vi "MGL_relativePath_cls.vi"(8 "name of main source folder [BIN]":string="BIN") -> (1 "mode":T1, 2 "Path":path)   [LabVIEW 2018]
uses:
  MGL_relativePathMode.ctl
panel:
  # "Relative Path.vi\n\nRitorna il path della directory dov'e' stato salvato, indipendentemente se chiamato da un eseguibile o no (VI di LabVIEW).\nUsando questo VI  per creare i path dei vari file utili ad un applicazione, non sarà poi necessario \nmodificare nulla creando l'eseguibile dell'applicazine.\n\nSe il VI viene salvato all'interno di directory che si trovano sotto una \"BIN\", ritornera' il path subito \"sopra\" la \"BIN\".\n - es \"C:\\app\\bin\\uno\\due\\tre\\Path.vi\"  ritornerà  \"c:\\app\"\nLo stesso vale se al posto di BIN si usano nomi che iniziano per BIN ( BINARY, BINS ...)\n\nCopyright (C) 2003 Alessandro Ricco - ale914@ilvg.it\n\n                                        Visita \"Italian LabVIEW user Group\" - www.ilvg.it\n\n\nThis library is free software; you can redistribute it and/or\nmodify it under the terms of the GNU Lesser General Public\nLicense as published by the Free Software Foundation; either\nversion 2.1 of the License, or (at your option) any later version.\nThis library is distributed in the hope that it will be useful,\nbut WITHOUT ANY WARRANTY; without even the implied warranty of\nMERCHANTABILITY or FITNESS FOR A PARTICULAR PURPOSE. See the GNU\nLesser General Public License for more details.\nYou should have received a copy of the GNU Lesser General Public\nLicense along with this library; if not, write to the Free Software\nFoundation, Inc., 59 Temple Place, Suite 330, Boston, MA 02111-1307 USA"
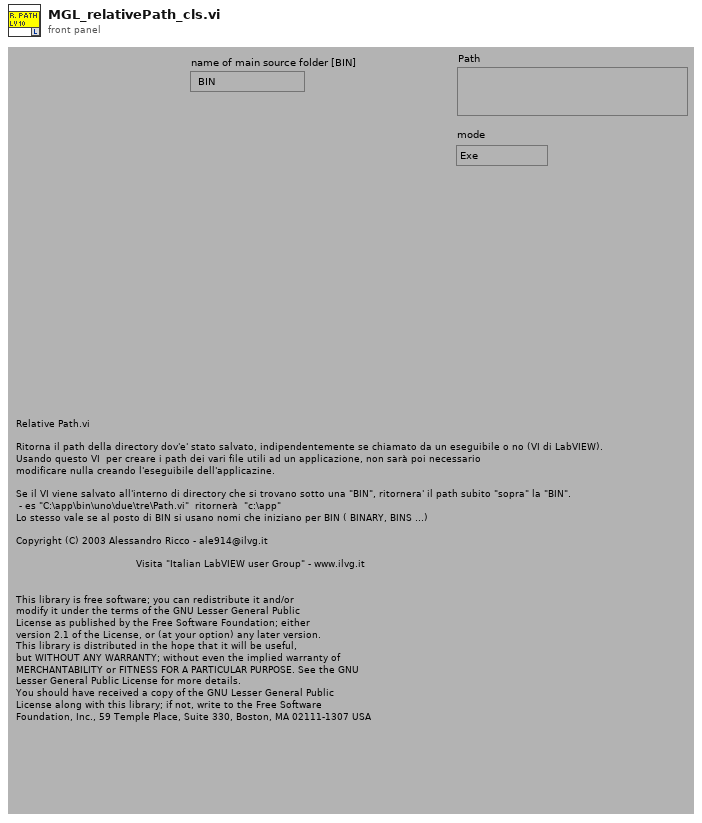
[diagram p1: front panel]
types:
  T1 = typedef "MGL_RelativePathMode.ctl" = enum16{"Exe", "LabVIEW"}
  T2 = typedef "MGL_relativePathMode.ctl" = enum16{"Exe", "LabVIEW"}
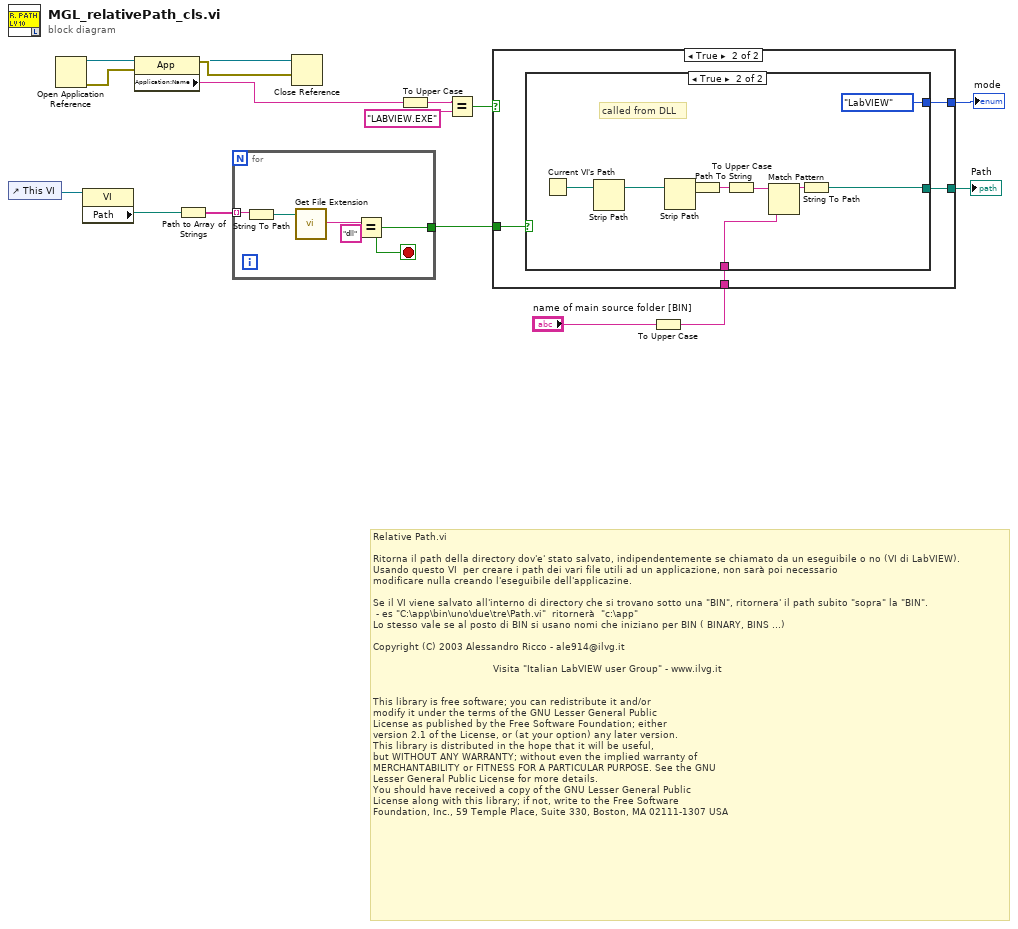
[diagram p0: block diagram]
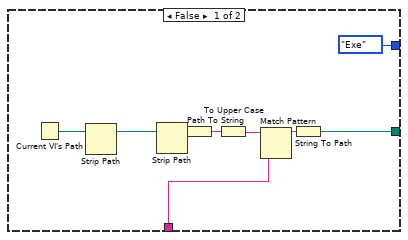
[diagram p2: hidden frame]
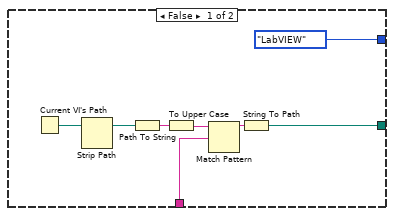
[diagram p3: hidden frame]
diagram:
  # "Relative Path.vi\n\nRitorna il path della directory dov'e' stato salvato, indipendentemente se chiamato da un eseguibile o no (VI di LabVIEW).\nUsando questo VI  per creare i path dei vari file utili ad un applicazione, non sarà poi necessario \nmodificare nulla creando l'eseguibile dell'applicazine.\n\nSe il VI viene salvato all'interno di directory che si trovano sotto una \"BIN\", ritornera' il path subito \"sopra\" la \"BIN\".\n - es \"C:\\app\\bin\\uno\\due\\tre\\Path.vi\"  ritornerà  \"c:\\app\"\nLo stesso vale se al posto di BIN si usano nomi che iniziano per BIN ( BINARY, BINS ...)\n\nCopyright (C) 2003 Alessandro Ricco - ale914@ilvg.it\n\n                                        Visita \"Italian LabVIEW user Group\" - www.ilvg.it\n\n\nThis library is free software; you can redistribute it and/or\nmodify it under the terms of the GNU Lesser General Public\nLicense as published by the Free Software Foundation; either\nversion 2.1 of the License, or (at your option) any later version.\nThis library is distributed in the hope that it will be useful,\nbut WITHOUT ANY WARRANTY; without even the implied warranty of\nMERCHANTABILITY or FITNESS FOR A PARTICULAR PURPOSE. See the GNU\nLesser General Public License for more details.\nYou should have received a copy of the GNU Lesser General Public\nLicense along with this library; if not, write to the Free Software\nFoundation, Inc., 59 Temple Place, Suite 330, Boston, MA 02111-1307 USA"
  n1 = control-ref of="This VI"() -> (w5:refnum<vi>)
  n2 = Open Application Reference() -> (0:w15:errorcluster, 3:w12:refnum<vi>)  [unwired: 1 in, 3 out]
  n3 = property class="VI"(reference=w5) -> ("Path"=w4:path)  [unwired: 1 in, 2 out]
  n4 = property class="App"(reference=w12, error in=w15) -> (reference out=w13:refnum<vi>, error out=w14:errorcluster, "Application:Name"=w7:string)
  n5 = Path to Array of Strings(0:w4) -> (2:w3:string[])  [unwired: 1 out]
  n6 = for {
    tunnel: w3 -> [w21] mode=indexing
    tunnel: [w17] -> w1
    stop <- w17 stop-if-true
    n7 = String To Path(string=w21) -> (path=w20:path)
    n8 = call <vilib>:"Get File Extension.vi"("file"=w20) -> ("lowercase file extension"=w19:string)  [unwired: 6 in, 4 out]
    n9 = Equal?(x=w19, y="dll") -> (x = y?=w17:bool)
  }
  n10 = Close Reference(reference=w13, error in (no error)=w14) -> ()  [unwired: 1 out]
  n11 = To Upper Case(1:w7) -> (0:w6:string)
  n12 = Equal?(x=w6, y="LABVIEW.EXE") -> (x = y?=w2:bool)
  n13 = To Upper Case(1:"name of main source folder [BIN]") -> (0:w8:string)
  n14 = case shown="True" w2 {
    tunnel: [w24 w34] -> w11
    tunnel: [MGL_RelativePathMode."Exe" ("mode") w33] -> w10
    tunnel: w8 -> [w22 w32]
    tunnel: w1 -> [_ w31]
    frame False {
      n15 = Current VI's Path() -> (path=w25:path)
      n16 = Strip Path(path=w25) -> (stripped path=w29:path)  [unwired: 1 out]
      n17 = Strip Path(path=w29) -> (stripped path=w30:path)  [unwired: 1 out]
      n18 = Path To String(path=w30) -> (string=w26:string)
      n19 = To Upper Case(1:w26) -> (0:w27:string)
      n20 = Match Pattern(string=w27, regular expression=w22) -> (before substring=w28:string)  [unwired: 4 out]
      n21 = String To Path(string=w28) -> (path=w24:path)
    }
    frame True {
      n22 = case shown="True" w31 {
        tunnel: [w38 w44] -> w34
        tunnel: [MGL_RelativePathMode."LabVIEW" ("mode") MGL_relativePathMode."LabVIEW" ("mode")] -> w33
        tunnel: w32 -> [w35 w45]
        frame False {
          n23 = Current VI's Path() -> (path=w37:path)
          n24 = Strip Path(path=w37) -> (stripped path=w39:path)  [unwired: 1 out]
          n25 = Path To String(path=w39) -> (string=w42:string)
          n26 = To Upper Case(1:w42) -> (0:w41:string)
          n27 = Match Pattern(string=w41, regular expression=w35) -> (before substring=w40:string)  [unwired: 4 out]
          n28 = String To Path(string=w40) -> (path=w38:path)
        }
        frame True {
          # "called from DLL"
          n29 = Current VI's Path() -> (path=w46:path)
          n30 = Strip Path(path=w46) -> (stripped path=w50:path)  [unwired: 1 out]
          n31 = Strip Path(path=w50) -> (stripped path=w51:path)  [unwired: 1 out]
          n32 = Path To String(path=w51) -> (string=w47:string)
          n33 = To Upper Case(1:w47) -> (0:w48:string)
          n34 = Match Pattern(string=w48, regular expression=w45) -> (before substring=w49:string)  [unwired: 4 out]
          n35 = String To Path(string=w49) -> (path=w44:path)
        }
      }
    }
  }
  "Path" <- w11
  "mode" <- w10
